vi "Immediate Minimums for Angle.vi"(9 "Power @ parallel to ground":dbl, 10 "Input":dbl, 11 "Angle":dbl) -> (3 "Output":dbl)   [LabVIEW 2018]
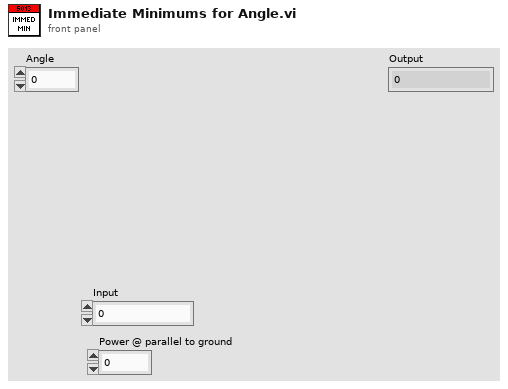
[diagram p1: front panel]
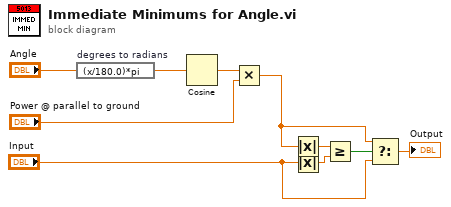
[diagram p0: block diagram]
diagram:
  n1 = expression code="(x/180.0)*pi" "degrees to radians"("Angle") -> (w10:dbl)
  n2 = Cosine(x=w10) -> (cos(x)=w9:dbl)
  n3 = Multiply(x=w9, y="Power @ parallel to ground") -> (x*y=w3:dbl)
  n4 = Absolute Value(x=w3) -> (abs(x)=w6:dbl)
  n5 = Absolute Value(x="Input") -> (abs(x)=w5:dbl)
  n6 = Greater Or Equal?(x=w6, y=w5) -> (x >= y?=w4:bool)
  n7 = Select(t=w3, s=w4, f="Input") -> (s? t:f=→"Output":dbl)
